vi "Scale Axes.vi"(8 "Axis 3 (throttle)":dbl, 10 "Axis 2 (y)":dbl, 11 "Axis 1 (x)":dbl) -> (2 "Scaled y":dbl, 3 "Scaled x":dbl)   [LabVIEW 2012]
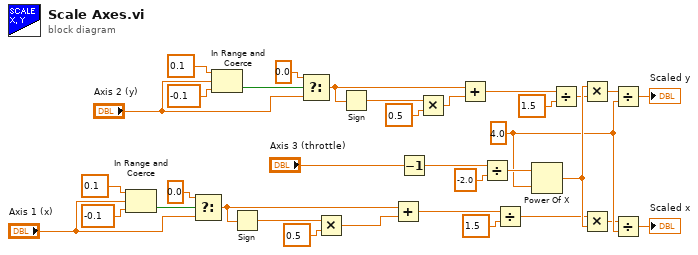
[diagram p0: block diagram]
diagram:
  w29 = 4.0 ("y")
  n1 = In Range and Coerce(upper limit=0.1, x="Axis 1 (x)", lower limit=-0.1) -> (In Range?=w6:bool)  [unwired: 1 out]
  n2 = Select(t=0.0, s=w6, f="Axis 1 (x)") -> (s? t:f=w4:dbl)
  n3 = In Range and Coerce(upper limit=0.1, x="Axis 2 (y)", lower limit=-0.1) -> (In Range?=w17:bool)  [unwired: 1 out]
  n4 = Sign(1:w4) -> (0:w11:dbl)
  n5 = Select(t=0.0, s=w17, f="Axis 2 (y)") -> (s? t:f=w14:dbl)
  n6 = Multiply(x=w11, y=0.5) -> (x*y=w10:dbl)
  n7 = Sign(1:w14) -> (0:w22:dbl)
  n8 = Add(x=w4, y=w10) -> (x+y=w13:dbl)
  n9 = Decrement(x="Axis 3 (throttle)") -> (x-1=w33:dbl)
  n10 = Multiply(x=w22, y=0.5) -> (x*y=w21:dbl)
  n11 = Add(x=w14, y=w21) -> (x+y=w24:dbl)
  n12 = Divide(x=w33, y=-2.0) -> (x/y=w31:dbl)
  n13 = Divide(x=w13, y=1.5) -> (x/y=w1:dbl)
  n14 = Power Of X(1:w29, 2:w31) -> (0:w30:dbl)
  n15 = Divide(x=w24, y=1.5) -> (x/y=w3:dbl)
  n16 = Multiply(x=w30, y=w3) -> (x*y=w27:dbl)
  n17 = Multiply(x=w1, y=w30) -> (x*y=w28:dbl)
  n18 = Divide(x=w27, y=w29) -> (x/y=→"Scaled y":dbl)
  n19 = Divide(x=w28, y=w29) -> (x/y=→"Scaled x":dbl)
